vi "ReplaceQueData.vi"(8 "ErrorArray":errorcluster[](array[cluster]), 10 "QueData":variant) -> (0 "ErrorArray 2":errorcluster[](array[cluster]))   [LabVIEW 2014, in "Bus_class.lvlib" / "Bus.lvclass"]
uses:
  Bus.lvclass
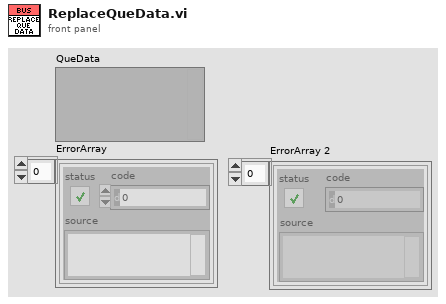
[diagram p1: front panel]
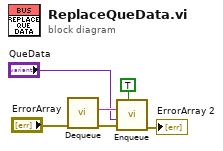
[diagram p0: block diagram]
diagram:
  n1 = call "Dequeue.vi"("ErrorArray"="ErrorArray") -> ("ErrorArray"=w2:errorcluster[], "Msg"=w4:string)  [unwired: 8 in, 1 out]
  n2 = call "Enqueue.vi"("Priority (f)"=TRUE, "ErrorArray"=w2, "Data"="QueData", "Msg"=w4) -> ("ErrorArray"=→"ErrorArray 2":errorcluster[])  [unwired: 7 in]
